vi "Poll Pool.vi"(8 "error in (no error)":errorcluster, 11 "cRIO-CO2 in":refnum<class "cRIO-CO2.lvclass">) -> ()   [LabVIEW 2015, in "cRIO-Carbondioxide.lvlib" / "cRIO-CO2.lvlib" / "cRIO-CO2.lvclass"]
uses:
  cRIO-CO2.lvclass
panel:
  out "error out":errorcluster
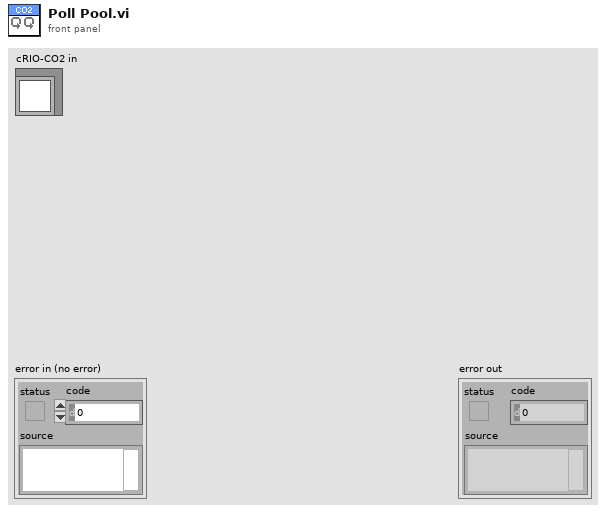
[diagram p1: front panel]
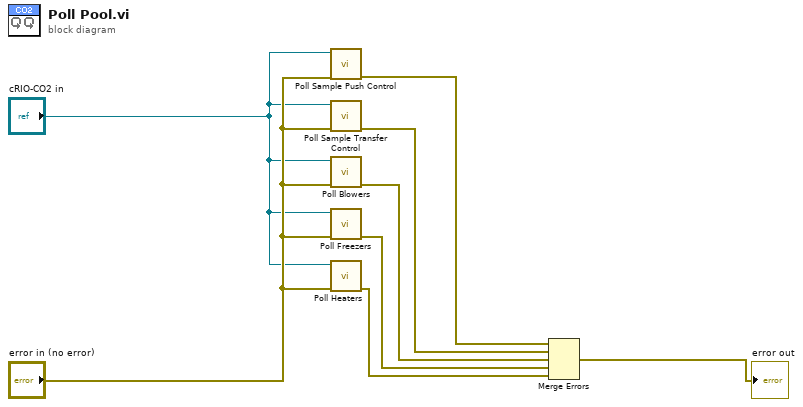
[diagram p0: block diagram]
diagram:
  n1 = call "Poll Sample Push Control.vi"("error in (no error)"="error in (no error)", "cRIO-CO2 in"="cRIO-CO2 in") -> ("error out"=w2:errorcluster)  [unwired: 8 in, 1 out]
  n2 = call "Poll Sample Transfer Control.vi"("error in (no error)"="error in (no error)", "cRIO-CO2 in"="cRIO-CO2 in") -> ("error out"=w3:errorcluster)  [unwired: 8 in, 1 out]
  n3 = call "Poll Blowers.vi"("error in (no error)"="error in (no error)", "cRIO-CO2 in"="cRIO-CO2 in") -> ("error IO"=w4:errorcluster)  [unwired: 9 in]
  n4 = call "Poll Freezers.vi"("error in (no error)"="error in (no error)", "cRIO-CO2 in"="cRIO-CO2 in") -> ("error out"=w5:errorcluster)  [unwired: 9 in]
  n5 = call "Poll Heaters.vi"("error in (no error)"="error in (no error)", "cRIO-CO2 in"="cRIO-CO2 in") -> ("error out"=w6:errorcluster)  [unwired: 9 in]
  n6 = Merge Errors(w2, w3, w4, w5, w6) -> (→"error out":errorcluster)
